vi "destroyHWEvents.vi"(8 "error in (no error)":errorcluster, 11 "HWControllerEvents in":refnum<class "HWControllerEvents.lvclass">) -> (0 "error out":errorcluster, 3 "HWControllerEvents out":refnum<class "HWControllerEvents.lvclass">)   [LabVIEW 2011, in "Hardware.lvlib" / "HWControllers.lvlib" / "HWControllerEvents.lvclass"]
doc: "HWController Events Destroy.\n\nAfter closing everything we destroy the events we were using to return the memory to the computer."
uses:
  HWControllerEvents.lvclass
  HWControllers.lvlib
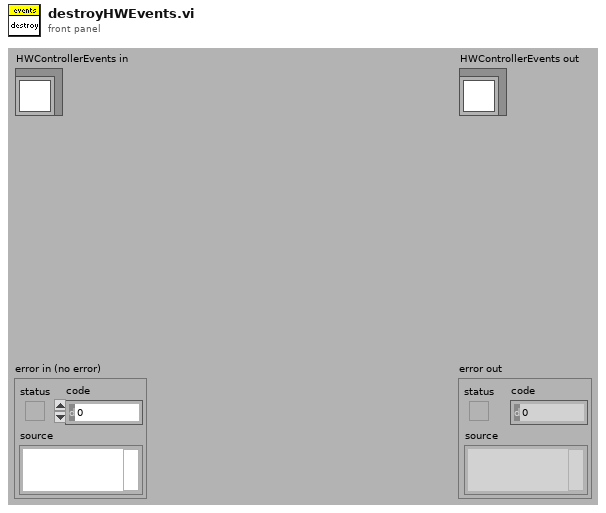
[diagram p1: front panel]
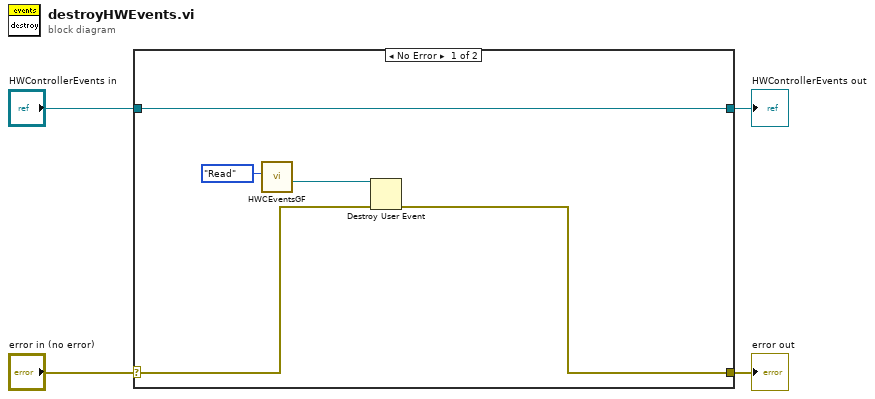
[diagram p0: block diagram]
diagram:
  n1 = case shown="No Error" "error in (no error)" {
    selector: "error in (no error)" -> [w8 w11]
    tunnel: [w7 w11] -> w3
    tunnel: [w9 w10] -> w1
    tunnel: "HWControllerEvents in" -> [w9 w10]
    frame No Error {
      n2 = call "HWCEventsGF.vi"("Action"=enum16{"Write", "Read"}."Read") -> ("HWCEvent"=w6:refnum<user-event>)  [unwired: 10 in]
      n3 = Destroy User Event(user event=w6, error in=w8) -> (error out=w7:errorcluster)
    }
    frame Error {
    }
  }
  "error out" <- w3
  "HWControllerEvents out" <- w1
